vi "Get Channel Attribute Double Wrapper.vi"(0 "Task map in":map{string, refnum<k21>}(c390), 5 "Message Data in":T2, 11 "error in (no error)":errorcluster) -> (4 "Task map out":map{string, refnum<k21>}(c390), 6 "Message Data out":T1, 15 "error out":errorcluster)   [LabVIEW 2021, in "NI DAQmx_wrapper.lvlib"]
uses:
  NI DAQmx_wrapper.lvlib
  NI DAQmx_server/RPC Messages/nidaqmx_grpc_GetChanAttributeDoubleRequest.ctl
  NI DAQmx_server/RPC Messages/nidevice_grpc_Session_session/nidevice_grpc_Session_session.lvclass
  NI DAQmx_server/RPC Messages/nidaqmx_grpc_GetChanAttributeDoubleRequest_attribute_enum/nidaqmx_grpc_GetChanAttributeDoubleRequest_attribute_enum.lvclass
  NI DAQmx_server/RPC Messages/nidevice_grpc_Session.ctl
  NI DAQmx_server/RPC Messages/nidaqmx_grpc_GetChanAttributeDoubleResponse.ctl
  NI DAQmx_server/RPC Messages/nidaqmx_grpc_GetChanAttributeDoubleRequest_attribute_enum/nidaqmx_grpc_GetChanAttributeDoubleRequest_attribute_enum.lvclass/nidaqmx_grpc_GetChanAttributeDoubleRequest_attribute_enum.ctl
  NI DAQmx_server/RPC Messages/nidevice_grpc_Session_session/nidevice_grpc_Session_session.lvclass/nidevice_grpc_Session_session.ctl
  <resource>/objmgr/daqmx.rc
  NI DAQmx_server/NI DAQmx_server.lvlib
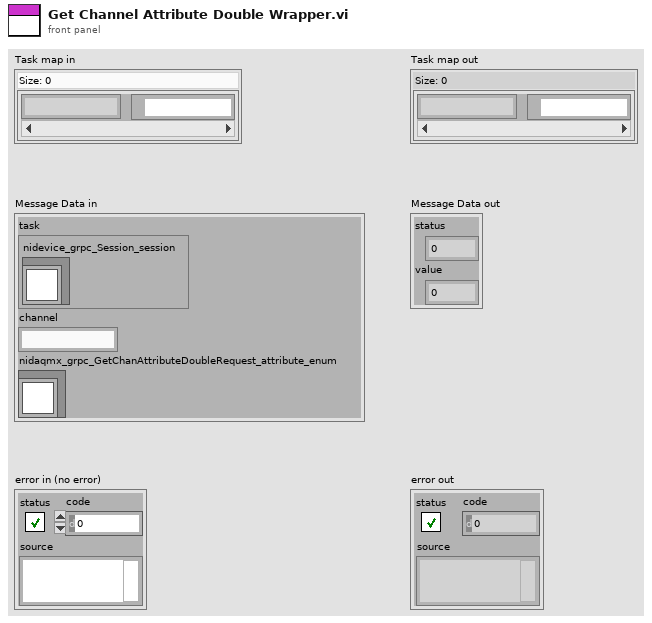
[diagram p1: front panel]
types:
  T1 = typedef "NI DAQmx_server.lvlib/nidaqmx_grpc_GetChanAttributeDoubleResponse.ctl" = cluster{"status":i32, "value":dbl}
  T2 = typedef "NI DAQmx_server.lvlib/nidaqmx_grpc_GetChanAttributeDoubleRequest.ctl" = cluster{"task":T3, "channel":string, "nidaqmx_grpc_GetChanAttributeDoubleRequest_attribute_enum":refnum<class "nidaqmx_grpc_GetChanAttributeDoubleRequest_attribute_enum.lvclass">}
  T3 = typedef "NI DAQmx_server.lvlib/nidevice_grpc_Session.ctl" = cluster{"nidevice_grpc_Session_session":refnum<class "nidevice_grpc_Session_session.lvclass">}
  T4 = typedef "NI DAQmx_server.lvlib/nidaqmx_grpc_ChannelDoubleAttribute.ctl" = enum32{"CHANNEL_DOUBLE_ATTRIBUTE_UNSPECIFIED", "CHANNEL_ATTRIBUTE_AI_IMPEDANCE", "CHANNEL_ATTRIBUTE_AI_AC_EXCIT_FREQ", "CHANNEL_ATTRIBUTE_AO_GAIN", "CHANNEL_ATTRIBUTE_AO_LOAD_IMPEDANCE", "CHANNEL_ATTRIBUTE_CI_FREQ_MEAS_TIME", "CHANNEL_ATTRIBUTE_CO_PULSE_FREQ_INITIAL_DELAY", "CHANNEL_ATTRIBUTE_AI_ACCEL_SENSITIVITY", "CHANNEL_ATTRIBUTE_AI_FREQ_HYST", "CHANNEL_ATTRIBUTE_AI_FREQ_THRESH_VOLTAGE", "CHANNEL_ATTRIBUTE_CI_ANG_ENCODER_INITIAL_ANGLE", "CHANNEL_ATTRIBUTE_CI_ENCODER_Z_INDEX_VAL", "CHANNEL_ATTRIBUTE_AI_RVDT_SENSITIVITY", "CHANNEL_ATTRIBUTE_CI_LIN_ENCODER_DIST_PER_PULSE", "CHANNEL_ATTRIBUTE_CI_LIN_ENCODER_INITIAL_POS", "CHANNEL_ATTRIBUTE_AI_LVDT_SENSITIVITY", "CHANNEL_ATTRIBUTE_AI_STRAIN_GAGE_GAGE_FACTOR", "CHANNEL_ATTRIBUTE_AI_STRAIN_GAGE_POISSON_RATIO", "CHANNEL_ATTRIBUTE_AI_RTD_A", "CHANNEL_ATTRIBUTE_AI_RTD_B", "CHANNEL_ATTRIBUTE_AI_RTD_C", "CHANNEL_ATTRIBUTE_AI_RTD_R0", "CHANNEL_ATTRIBUTE_AI_THRMCPL_CJC_VAL", "CHANNEL_ATTRIBUTE_AI_THRMSTR_R1", "CHANNEL_ATTRIBUTE_CO_PULSE_DUTY_CYC", "CHANNEL_ATTRIBUTE_CO_PULSE_FREQ", "CHANNEL_ATTRIBUTE_AO_MAX", "CHANNEL_ATTRIBUTE_AO_MIN", "CHANNEL_ATTRIBUTE_AO_OUTPUT_IMPEDANCE", "CHANNEL_ATTRIBUTE_AI_MICROPHONE_SENSITIVITY", "CHANNEL_ATTRIBUTE_AI_RESOLUTION", "CHANNEL_ATTRIBUTE_AI_MAX", "CHANNEL_ATTRIBUTE_AI_MIN", "CHANNEL_ATTRIBUTE_AI_BRIDGE_NOM_RESISTANCE", "CHANNEL_ATTRIBUTE_AI_BRIDGE_INITIAL_VOLTAGE", "CHANNEL_ATTRIBUTE_AI_LEAD_WIRE_RESISTANCE", "CHANNEL_ATTRIBUTE_AI_CURRENT_SHUNT_RESISTANCE", "CHANNEL_ATTRIBUTE_AI_EXCIT_VAL", "CHANNEL_ATTRIBUTE_AI_ATTEN", "CHANNEL_ATTRIBUTE_AI_LOWPASS_CUTOFF_FREQ", "CHANNEL_ATTRIBUTE_AI_HIGHPASS_CUTOFF_FREQ", "CHANNEL_ATTRIBUTE_AI_BANDPASS_CENTER_FREQ", "CHANNEL_ATTRIBUTE_AI_BANDPASS_WIDTH", "CHANNEL_ATTRIBUTE_AI_NOTCH_CENTER_FREQ", "CHANNEL_ATTRIBUTE_AI_NOTCH_WIDTH", "CHANNEL_ATTRIBUTE_AI_RNG_HIGH", "CHANNEL_ATTRIBUTE_AI_RNG_LOW", "CHANNEL_ATTRIBUTE_AI_GAIN", "CHANNEL_ATTRIBUTE_AO_RESOLUTION", "CHANNEL_ATTRIBUTE_AO_DAC_RNG_LOW", "CHANNEL_ATTRIBUTE_AO_DAC_RNG_HIGH", "CHANNEL_ATTRIBUTE_AO_DAC_REF_VAL", "CHANNEL_ATTRIBUTE_AI_EXCIT_ACTUAL_VAL", "CHANNEL_ATTRIBUTE_AI_LOWPASS_SWITCH_CAP_EXT_CLK_FREQ", "CHANNEL_ATTRIBUTE_CI_MAX", "CHANNEL_ATTRIBUTE_CI_MIN", "CHANNEL_ATTRIBUTE_CI_CTR_TIMEBASE_RATE", "CHANNEL_ATTRIBUTE_CO_PULSE_HIGH_TIME", "CHANNEL_ATTRIBUTE_CO_PULSE_LOW_TIME", "CHANNEL_ATTRIBUTE_CO_PULSE_TIME_INITIAL_DELAY", "CHANNEL_ATTRIBUTE_CO_CTR_TIMEBASE_RATE", "CHANNEL_ATTRIBUTE_AI_THRMSTR_A", "CHANNEL_ATTRIBUTE_AI_THRMSTR_C", "CHANNEL_ATTRIBUTE_AI_THRMSTR_B", "CHANNEL_ATTRIBUTE_CI_PERIOD_MEAS_TIME", "CHANNEL_ATTRIBUTE_AI_BRIDGE_SHUNT_CAL_GAIN_ADJUST", "CHANNEL_ATTRIBUTE_DI_DIG_FLTR_MIN_PULSE_WIDTH", "CHANNEL_ATTRIBUTE_CI_FREQ_DIG_FLTR_MIN_PULSE_WIDTH", "CHANNEL_ATTRIBUTE_CI_FREQ_DIG_FLTR_TIMEBASE_RATE", "CHANNEL_ATTRIBUTE_CI_PERIOD_DIG_FLTR_MIN_PULSE_WIDTH", "CHANNEL_ATTRIBUTE_CI_PERIOD_DIG_FLTR_TIMEBASE_RATE", "CHANNEL_ATTRIBUTE_CI_COUNT_EDGES_COUNT_DIR_DIG_FLTR_MIN_PULSE_WIDTH", "CHANNEL_ATTRIBUTE_CI_COUNT_EDGES_COUNT_DIR_DIG_FLTR_TIMEBASE_RATE", "CHANNEL_ATTRIBUTE_CI_COUNT_EDGES_DIG_FLTR_MIN_PULSE_WIDTH", "CHANNEL_ATTRIBUTE_CI_COUNT_EDGES_DIG_FLTR_TIMEBASE_RATE", "CHANNEL_ATTRIBUTE_CI_ENCODER_A_INPUT_DIG_FLTR_MIN_PULSE_WIDTH", "CHANNEL_ATTRIBUTE_CI_ENCODER_A_INPUT_DIG_FLTR_TIMEBASE_RATE", "CHANNEL_ATTRIBUTE_CI_ENCODER_B_INPUT_DIG_FLTR_MIN_PULSE_WIDTH", "CHANNEL_ATTRIBUTE_CI_ENCODER_B_INPUT_DIG_FLTR_TIMEBASE_RATE", "CHANNEL_ATTRIBUTE_CI_ENCODER_Z_INPUT_DIG_FLTR_MIN_PULSE_WIDTH", "CHANNEL_ATTRIBUTE_CI_ENCODER_Z_INPUT_DIG_FLTR_TIMEBASE_RATE", "CHANNEL_ATTRIBUTE_CI_PULSE_WIDTH_DIG_FLTR_MIN_PULSE_WIDTH", "CHANNEL_ATTRIBUTE_CI_PULSE_WIDTH_DIG_FLTR_TIMEBASE_RATE", "CHANNEL_ATTRIBUTE_CI_TWO_EDGE_SEP_FIRST_DIG_FLTR_MIN_PULSE_WIDTH", "CHANNEL_ATTRIBUTE_CI_TWO_EDGE_SEP_FIRST_DIG_FLTR_TIMEBASE_RATE", "CHANNEL_ATTRIBUTE_CI_TWO_EDGE_SEP_SECOND_DIG_FLTR_MIN_PULSE_WIDTH", "CHANNEL_ATTRIBUTE_CI_TWO_EDGE_SEP_SECOND_DIG_FLTR_TIMEBASE_RATE", "CHANNEL_ATTRIBUTE_CI_SEMI_PERIOD_DIG_FLTR_MIN_PULSE_WIDTH", "CHANNEL_ATTRIBUTE_CI_SEMI_PERIOD_DIG_FLTR_TIMEBASE_RATE", "CHANNEL_ATTRIBUTE_AI_SOUND_PRESSURE_MAX_SOUND_PRESSURE_LVL", "CHANNEL_ATTRIBUTE_AO_DAC_OFFSET_VAL", "CHANNEL_ATTRIBUTE_CI_CTR_TIMEBASE_DIG_FLTR_MIN_PULSE_WIDTH", "CHANNEL_ATTRIBUTE_CI_CTR_TIMEBASE_DIG_FLTR_TIMEBASE_RATE", "CHANNEL_ATTRIBUTE_CO_CTR_TIMEBASE_DIG_FLTR_MIN_PULSE_WIDTH", "CHANNEL_ATTRIBUTE_CO_CTR_TIMEBASE_DIG_FLTR_TIMEBASE_RATE", "CHANNEL_ATTRIBUTE_AI_VOLTAGE_DB_REF", "CHANNEL_ATTRIBUTE_AI_SOUND_PRESSURE_DB_REF", "CHANNEL_ATTRIBUTE_AI_ACCEL_DB_REF", "CHANNEL_ATTRIBUTE_AO_FUNC_GEN_FREQ", "CHANNEL_ATTRIBUTE_AO_FUNC_GEN_AMPLITUDE", "CHANNEL_ATTRIBUTE_AO_FUNC_GEN_OFFSET", "CHANNEL_ATTRIBUTE_AO_FUNC_GEN_SQUARE_DUTY_CYCLE", "CHANNEL_ATTRIBUTE_AO_VOLTAGE_CURRENT_LIMIT", "CHANNEL_ATTRIBUTE_AO_FUNC_GEN_FM_DEVIATION", "CHANNEL_ATTRIBUTE_DO_OVERCURRENT_LIMIT", "CHANNEL_ATTRIBUTE_DO_OVERCURRENT_REENABLE_PERIOD", "CHANNEL_ATTRIBUTE_AI_PROBE_ATTEN", "CHANNEL_ATTRIBUTE_AI_DC_OFFSET", "CHANNEL_ATTRIBUTE_AI_EDDY_CURRENT_PROX_PROBE_SENSITIVITY", "CHANNEL_ATTRIBUTE_DI_DIG_FLTR_TIMEBASE_RATE", "CHANNEL_ATTRIBUTE_CI_PULSE_FREQ_DIG_FLTR_MIN_PULSE_WIDTH", "CHANNEL_ATTRIBUTE_CI_PULSE_FREQ_DIG_FLTR_TIMEBASE_RATE", "CHANNEL_ATTRIBUTE_CI_PULSE_TIME_DIG_FLTR_MIN_PULSE_WIDTH", "CHANNEL_ATTRIBUTE_CI_PULSE_TIME_DIG_FLTR_TIMEBASE_RATE", "CHANNEL_ATTRIBUTE_CI_PULSE_TICKS_DIG_FLTR_MIN_PULSE_WIDTH", "CHANNEL_ATTRIBUTE_CI_PULSE_TICKS_DIG_FLTR_TIMEBASE_RATE", "CHANNEL_ATTRIBUTE_AI_BRIDGE_SHUNT_CAL_SHUNT_CAL_A_RESISTANCE", "CHANNEL_ATTRIBUTE_AI_BRIDGE_SHUNT_CAL_SHUNT_CAL_A_ACTUAL_RESISTANCE", "CHANNEL_ATTRIBUTE_AI_BRIDGE_SHUNT_CAL_SHUNT_CAL_B_RESISTANCE", "CHANNEL_ATTRIBUTE_AI_BRIDGE_SHUNT_CAL_SHUNT_CAL_B_ACTUAL_RESISTANCE", "CHANNEL_ATTRIBUTE_AI_FORCE_IEPE_SENSOR_SENSITIVITY", "CHANNEL_ATTRIBUTE_AI_BRIDGE_INITIAL_RATIO", "CHANNEL_ATTRIBUTE_AI_BRIDGE_TWO_POINT_LIN_FIRST_ELECTRICAL_VAL", "CHANNEL_ATTRIBUTE_AI_BRIDGE_TWO_POINT_LIN_FIRST_PHYSICAL_VAL", "CHANNEL_ATTRIBUTE_AI_BRIDGE_TWO_POINT_LIN_SECOND_ELECTRICAL_VAL", "CHANNEL_ATTRIBUTE_AI_BRIDGE_TWO_POINT_LIN_SECOND_PHYSICAL_VAL", "CHANNEL_ATTRIBUTE_CI_COUNT_EDGES_COUNT_RESET_DIG_FLTR_MIN_PULSE_WIDTH", "CHANNEL_ATTRIBUTE_CI_COUNT_EDGES_COUNT_RESET_DIG_FLTR_TIMEBASE_RATE", "CHANNEL_ATTRIBUTE_AI_THRMCPL_LEAD_OFFSET_VOLTAGE", "CHANNEL_ATTRIBUTE_AI_FILTER_DELAY", "CHANNEL_ATTRIBUTE_AI_VELOCITY_IEPE_SENSOR_DB_REF", "CHANNEL_ATTRIBUTE_AI_VELOCITY_IEPE_SENSOR_SENSITIVITY", "CHANNEL_ATTRIBUTE_AI_ROSETTE_STRAIN_GAGE_ORIENTATION", "CHANNEL_ATTRIBUTE_AO_FILTER_DELAY_ADJUSTMENT", "CHANNEL_ATTRIBUTE_AI_FILTER_DELAY_ADJUSTMENT", "CHANNEL_ATTRIBUTE_AO_FILTER_DELAY", "CHANNEL_ATTRIBUTE_CI_DUTY_CYCLE_DIG_FLTR_MIN_PULSE_WIDTH", "CHANNEL_ATTRIBUTE_CI_DUTY_CYCLE_DIG_FLTR_TIMEBASE_RATE", "CHANNEL_ATTRIBUTE_CI_MAX_MEAS_PERIOD", "CHANNEL_ATTRIBUTE_CI_THRESH_VOLTAGE", "CHANNEL_ATTRIBUTE_AI_DIG_FLTR_LOWPASS_CUTOFF_FREQ", "CHANNEL_ATTRIBUTE_AI_DIG_FLTR_HIGHPASS_CUTOFF_FREQ", "CHANNEL_ATTRIBUTE_AI_DIG_FLTR_BANDPASS_CENTER_FREQ", "CHANNEL_ATTRIBUTE_AI_DIG_FLTR_BANDPASS_WIDTH", "CHANNEL_ATTRIBUTE_AI_DIG_FLTR_NOTCH_CENTER_FREQ", "CHANNEL_ATTRIBUTE_AI_DIG_FLTR_NOTCH_WIDTH", "CHANNEL_ATTRIBUTE_CI_VELOCITY_LIN_ENCODER_DIST_PER_PULSE", "CHANNEL_ATTRIBUTE_CI_VELOCITY_ENCODER_A_INPUT_DIG_FLTR_MIN_PULSE_WIDTH", "CHANNEL_ATTRIBUTE_CI_VELOCITY_ENCODER_A_INPUT_DIG_FLTR_TIMEBASE_RATE", "CHANNEL_ATTRIBUTE_CI_VELOCITY_ENCODER_B_INPUT_DIG_FLTR_MIN_PULSE_WIDTH", "CHANNEL_ATTRIBUTE_CI_VELOCITY_ENCODER_B_INPUT_DIG_FLTR_TIMEBASE_RATE", "CHANNEL_ATTRIBUTE_CI_VELOCITY_MEAS_TIME", "CHANNEL_ATTRIBUTE_CI_COUNT_EDGES_GATE_DIG_FLTR_MIN_PULSE_WIDTH", "CHANNEL_ATTRIBUTE_CI_COUNT_EDGES_GATE_DIG_FLTR_TIMEBASE_RATE", "CHANNEL_ATTRIBUTE_AI_ACCEL_CHARGE_SENSITIVITY", "CHANNEL_ATTRIBUTE_AI_ACCEL_4_WIRE_DC_VOLTAGE_SENSITIVITY", "CHANNEL_ATTRIBUTE_AI_DATA_XFER_MAX_RATE", "CHANNEL_ATTRIBUTE_AI_SENSOR_POWER_VOLTAGE", "CHANNEL_ATTRIBUTE_AI_FILTER_FREQ", "CHANNEL_ATTRIBUTE_AI_INPUT_LIMITS_FAULT_DETECT_UPPER_LIMIT", "CHANNEL_ATTRIBUTE_AI_INPUT_LIMITS_FAULT_DETECT_LOWER_LIMIT", "CHANNEL_ATTRIBUTE_CI_FREQ_THRESH_VOLTAGE", "CHANNEL_ATTRIBUTE_CI_FREQ_HYST", "CHANNEL_ATTRIBUTE_CI_PERIOD_THRESH_VOLTAGE", "CHANNEL_ATTRIBUTE_CI_PERIOD_HYST", "CHANNEL_ATTRIBUTE_CI_COUNT_EDGES_THRESH_VOLTAGE", "CHANNEL_ATTRIBUTE_CI_COUNT_EDGES_HYST", "CHANNEL_ATTRIBUTE_CI_COUNT_EDGES_COUNT_DIR_THRESH_VOLTAGE", "CHANNEL_ATTRIBUTE_CI_COUNT_EDGES_COUNT_DIR_HYST", "CHANNEL_ATTRIBUTE_CI_COUNT_EDGES_COUNT_RESET_THRESH_VOLTAGE", "CHANNEL_ATTRIBUTE_CI_COUNT_EDGES_COUNT_RESET_HYST", "CHANNEL_ATTRIBUTE_CI_COUNT_EDGES_GATE_THRESH_VOLTAGE", "CHANNEL_ATTRIBUTE_CI_COUNT_EDGES_GATE_HYST", "CHANNEL_ATTRIBUTE_CI_FILTER_FREQ", "CHANNEL_ATTRIBUTE_CI_FILTER_DELAY", "CHANNEL_ATTRIBUTE_AO_FUNC_GEN_START_PHASE", "CHANNEL_ATTRIBUTE_AO_COMMON_MODE_OFFSET", "CHANNEL_ATTRIBUTE_PWR_VOLTAGE_SETPOINT", "CHANNEL_ATTRIBUTE_PWR_CURRENT_SETPOINT"}
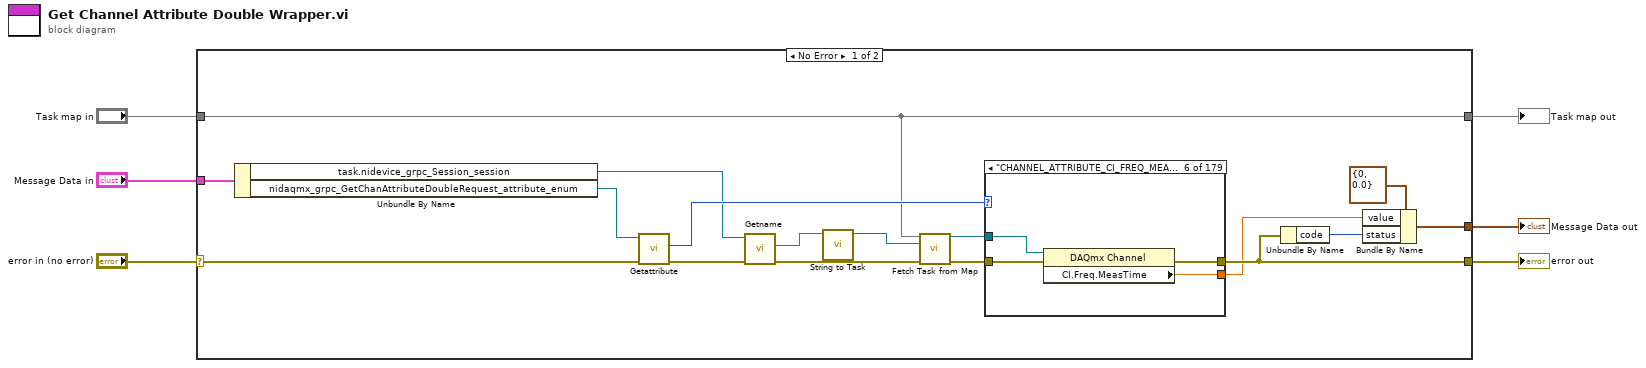
[diagram p0: block diagram]
diagram:
  n1 = case shown="No Error" "error in (no error)" {
    selector: "error in (no error)" -> [w22 w207]
    tunnel: [w10 w207] -> w5
    tunnel: "Task map in" -> [w13 w206]
    tunnel: [w13 w206] -> w3
    tunnel: "Message Data in" -> [w23 _]
    tunnel: [w7 _] -> w1
    frame No Error {
      n2 = Unbundle By Name(w23) -> ("task.nidevice_grpc_Session_session"=w14:refnum<class "nidevice_grpc_Session_session.lvclass">, "nidaqmx_grpc_GetChanAttributeDoubleRequest_attribute_enum"=w21:refnum<class "nidaqmx_grpc_GetChanAttributeDoubleRequest_attribute_enum.lvclass">)
      n3 = call "Getattribute.vi"("error in (no error)"=w22, "OneOfTemplate in"=w21) -> ("error out"=w16:errorcluster, "Get_Val"=w20:T4)  [unwired: 7 in, 1 out]
      n4 = call "Getname.vi"("error in (no error)"=w16, "OneOfTemplate in"=w14) -> ("error out"=w17:errorcluster, "Get_Val"=w19:string)  [unwired: 7 in, 1 out]
      n5 = call "String to Task.vi"("Get_Val"=w19) -> ("Refnum out"=w18:refnum<k21>)  [unwired: 10 in]
      n6 = call "Fetch Task from Map.vi"("Task map in"=w13, "Task in"=w18, "error in (no error)"=w17) -> ("Task out"=w12:refnum<k21>, "error out"=w15:errorcluster)  [unwired: 11 in]
      n7 = case shown="\"CHANNEL_ATTRIBUTE_CI_FREQ_MEAS_TIME\"" w20 {
        tunnel: w15 -> [w24 w25 w26 w27 w28 w32 w33 w34 w35 w36 w37 w38 w39 w40 w41 w42 w43 w44 w45 w46 w47 w48 w49 w50 w51 w52 w53 w54 w55 w56 w57 w58 w59 w60 w61 w62 w63 w64 w65 w66 w67 w68 w69 w70 w71 w72 w73 w74 w75 w76 w77 w78 w79 w80 w81 w82 w83 w84 w85 w86 w87 w88 w89 w90 w91 w92 w93 w94 w95 w96 w97 w98 w99 w100 w101 w102 w103 w104 w105 w106 w107 w108 w109 w110 w111 w112 w113 w114 w115 w116 w117 w118 w119 w120 w121 w122 w123 w124 w125 w126 w127 w128 w129 w130 w131 w132 w133 w134 w135 w136 w137 w138 w139 w140 w141 w142 w143 w144 w145 w146 w147 w148 w149 w150 w151 w152 w153 w154 w155 w156 w157 w158 w159 w160 w161 w162 w163 w164 w165 w166 w167 w168 w169 w170 w171 w172 w173 w174 w175 w176 w177 w178 w179 w180 w181 w182 w183 w184 w185 w186 w187 w188 w189 w190 w191 w192 w193 w194 w195 w196 w197 w198 w199 w200 w201 w202 w203 w204 w205]
        tunnel: [w24 w25 w26 w27 w28 w31 w33 w34 w35 w36 w37 w38 w39 w40 w41 w42 w43 w44 w45 w46 w47 w48 w49 w50 w51 w52 w53 w54 w55 w56 w57 w58 w59 w60 w61 w62 w63 w64 w65 w66 w67 w68 w69 w70 w71 w72 w73 w74 w75 w76 w77 w78 w79 w80 w81 w82 w83 w84 w85 w86 w87 w88 w89 w90 w91 w92 w93 w94 w95 w96 w97 w98 w99 w100 w101 w102 w103 w104 w105 w106 w107 w108 w109 w110 w111 w112 w113 w114 w115 w116 w117 w118 w119 w120 w121 w122 w123 w124 w125 w126 w127 w128 w129 w130 w131 w132 w133 w134 w135 w136 w137 w138 w139 w140 w141 w142 w143 w144 w145 w146 w147 w148 w149 w150 w151 w152 w153 w154 w155 w156 w157 w158 w159 w160 w161 w162 w163 w164 w165 w166 w167 w168 w169 w170 w171 w172 w173 w174 w175 w176 w177 w178 w179 w180 w181 w182 w183 w184 w185 w186 w187 w188 w189 w190 w191 w192 w193 w194 w195 w196 w197 w198 w199 w200 w201 w202 w203 w204 w205] -> w10
        tunnel: w12 -> [_ _ _ _ _ w30 _ _ _ _ _ _ _ _ _ _ _ _ _ _ _ _ _ _ _ _ _ _ _ _ _ _ _ _ _ _ _ _ _ _ _ _ _ _ _ _ _ _ _ _ _ _ _ _ _ _ _ _ _ _ _ _ _ _ _ _ _ _ _ _ _ _ _ _ _ _ _ _ _ _ _ _ _ _ _ _ _ _ _ _ _ _ _ _ _ _ _ _ _ _ _ _ _ _ _ _ _ _ _ _ _ _ _ _ _ _ _ _ _ _ _ _ _ _ _ _ _ _ _ _ _ _ _ _ _ _ _ _ _ _ _ _ _ _ _ _ _ _ _ _ _ _ _ _ _ _ _ _ _ _ _ _ _ _ _ _ _ _ _ _ _ _ _ _ _ _ _ _ _]
        tunnel: [_ _ _ _ _ w29 _ _ _ _ _ _ _ _ _ _ _ _ _ _ _ _ _ _ _ _ _ _ _ _ _ _ _ _ _ _ _ _ _ _ _ _ _ _ _ _ _ _ _ _ _ _ _ _ _ _ _ _ _ _ _ _ _ _ _ _ _ _ _ _ _ _ _ _ _ _ _ _ _ _ _ _ _ _ _ _ _ _ _ _ _ _ _ _ _ _ _ _ _ _ _ _ _ _ _ _ _ _ _ _ _ _ _ _ _ _ _ _ _ _ _ _ _ _ _ _ _ _ _ _ _ _ _ _ _ _ _ _ _ _ _ _ _ _ _ _ _ _ _ _ _ _ _ _ _ _ _ _ _ _ _ _ _ _ _ _ _ _ _ _ _ _ _ _ _ _ _ _ _] -> w8
        frame "CHANNEL_DOUBLE_ATTRIBUTE_UNSPECIFIED", Default {
        }
        frame "CHANNEL_ATTRIBUTE_AI_IMPEDANCE" {
        }
        frame "CHANNEL_ATTRIBUTE_AI_AC_EXCIT_FREQ" {
        }
        frame "CHANNEL_ATTRIBUTE_AO_GAIN" {
        }
        frame "CHANNEL_ATTRIBUTE_AO_LOAD_IMPEDANCE" {
        }
        frame "CHANNEL_ATTRIBUTE_CI_FREQ_MEAS_TIME" {
          n8 = property class="DAQmx Channel"(reference=w30, error in=w32) -> (error out=w31:errorcluster, "CI.Freq.MeasTime"=w29:dbl)  [unwired: 1 out]
        }
        frame "CHANNEL_ATTRIBUTE_CO_PULSE_FREQ_INITIAL_DELAY" {
        }
        frame "CHANNEL_ATTRIBUTE_AI_ACCEL_SENSITIVITY" {
        }
        frame "CHANNEL_ATTRIBUTE_AI_FREQ_HYST" {
        }
        frame "CHANNEL_ATTRIBUTE_AI_FREQ_THRESH_VOLTAGE" {
        }
        frame "CHANNEL_ATTRIBUTE_CI_ANG_ENCODER_INITIAL_ANGLE" {
        }
        frame "CHANNEL_ATTRIBUTE_CI_ENCODER_Z_INDEX_VAL" {
        }
        frame "CHANNEL_ATTRIBUTE_AI_RVDT_SENSITIVITY" {
        }
        frame "CHANNEL_ATTRIBUTE_CI_LIN_ENCODER_DIST_PER_PULSE" {
        }
        frame "CHANNEL_ATTRIBUTE_CI_LIN_ENCODER_INITIAL_POS" {
        }
        frame "CHANNEL_ATTRIBUTE_AI_LVDT_SENSITIVITY" {
        }
        frame "CHANNEL_ATTRIBUTE_AI_STRAIN_GAGE_GAGE_FACTOR" {
        }
        frame "CHANNEL_ATTRIBUTE_AI_STRAIN_GAGE_POISSON_RATIO" {
        }
        frame "CHANNEL_ATTRIBUTE_AI_RTD_A" {
        }
        frame "CHANNEL_ATTRIBUTE_AI_RTD_B" {
        }
        frame "CHANNEL_ATTRIBUTE_AI_RTD_C" {
        }
        frame "CHANNEL_ATTRIBUTE_AI_RTD_R0" {
        }
        frame "CHANNEL_ATTRIBUTE_AI_THRMCPL_CJC_VAL" {
        }
        frame "CHANNEL_ATTRIBUTE_AI_THRMSTR_R1" {
        }
        frame "CHANNEL_ATTRIBUTE_CO_PULSE_DUTY_CYC" {
        }
        frame "CHANNEL_ATTRIBUTE_CO_PULSE_FREQ" {
        }
        frame "CHANNEL_ATTRIBUTE_AO_MAX" {
        }
        frame "CHANNEL_ATTRIBUTE_AO_MIN" {
        }
        frame "CHANNEL_ATTRIBUTE_AO_OUTPUT_IMPEDANCE" {
        }
        frame "CHANNEL_ATTRIBUTE_AI_MICROPHONE_SENSITIVITY" {
        }
        frame "CHANNEL_ATTRIBUTE_AI_RESOLUTION" {
        }
        frame "CHANNEL_ATTRIBUTE_AI_MAX" {
        }
        frame "CHANNEL_ATTRIBUTE_AI_MIN" {
        }
        frame "CHANNEL_ATTRIBUTE_AI_BRIDGE_NOM_RESISTANCE" {
        }
        frame "CHANNEL_ATTRIBUTE_AI_BRIDGE_INITIAL_VOLTAGE" {
        }
        frame "CHANNEL_ATTRIBUTE_AI_LEAD_WIRE_RESISTANCE" {
        }
        frame "CHANNEL_ATTRIBUTE_AI_CURRENT_SHUNT_RESISTANCE" {
        }
        frame "CHANNEL_ATTRIBUTE_AI_EXCIT_VAL" {
        }
        frame "CHANNEL_ATTRIBUTE_AI_ATTEN" {
        }
        frame "CHANNEL_ATTRIBUTE_AI_LOWPASS_CUTOFF_FREQ" {
        }
        frame "CHANNEL_ATTRIBUTE_AI_HIGHPASS_CUTOFF_FREQ" {
        }
        frame "CHANNEL_ATTRIBUTE_AI_BANDPASS_CENTER_FREQ" {
        }
        frame "CHANNEL_ATTRIBUTE_AI_BANDPASS_WIDTH" {
        }
        frame "CHANNEL_ATTRIBUTE_AI_NOTCH_CENTER_FREQ" {
        }
        frame "CHANNEL_ATTRIBUTE_AI_NOTCH_WIDTH" {
        }
        frame "CHANNEL_ATTRIBUTE_AI_RNG_HIGH" {
        }
        frame "CHANNEL_ATTRIBUTE_AI_RNG_LOW" {
        }
        frame "CHANNEL_ATTRIBUTE_AI_GAIN" {
        }
        frame "CHANNEL_ATTRIBUTE_AO_RESOLUTION" {
        }
        frame "CHANNEL_ATTRIBUTE_AO_DAC_RNG_LOW" {
        }
        frame "CHANNEL_ATTRIBUTE_AO_DAC_RNG_HIGH" {
        }
        frame "CHANNEL_ATTRIBUTE_AO_DAC_REF_VAL" {
        }
        frame "CHANNEL_ATTRIBUTE_AI_EXCIT_ACTUAL_VAL" {
        }
        frame "CHANNEL_ATTRIBUTE_AI_LOWPASS_SWITCH_CAP_EXT_CLK_FREQ" {
        }
        frame "CHANNEL_ATTRIBUTE_CI_MAX" {
        }
        frame "CHANNEL_ATTRIBUTE_CI_MIN" {
        }
        frame "CHANNEL_ATTRIBUTE_CI_CTR_TIMEBASE_RATE" {
        }
        frame "CHANNEL_ATTRIBUTE_CO_PULSE_HIGH_TIME" {
        }
        frame "CHANNEL_ATTRIBUTE_CO_PULSE_LOW_TIME" {
        }
        frame "CHANNEL_ATTRIBUTE_CO_PULSE_TIME_INITIAL_DELAY" {
        }
        frame "CHANNEL_ATTRIBUTE_CO_CTR_TIMEBASE_RATE" {
        }
        frame "CHANNEL_ATTRIBUTE_AI_THRMSTR_A" {
        }
        frame "CHANNEL_ATTRIBUTE_AI_THRMSTR_C" {
        }
        frame "CHANNEL_ATTRIBUTE_AI_THRMSTR_B" {
        }
        frame "CHANNEL_ATTRIBUTE_CI_PERIOD_MEAS_TIME" {
        }
        frame "CHANNEL_ATTRIBUTE_AI_BRIDGE_SHUNT_CAL_GAIN_ADJUST" {
        }
        frame "CHANNEL_ATTRIBUTE_DI_DIG_FLTR_MIN_PULSE_WIDTH" {
        }
        frame "CHANNEL_ATTRIBUTE_CI_FREQ_DIG_FLTR_MIN_PULSE_WIDTH" {
        }
        frame "CHANNEL_ATTRIBUTE_CI_FREQ_DIG_FLTR_TIMEBASE_RATE" {
        }
        frame "CHANNEL_ATTRIBUTE_CI_PERIOD_DIG_FLTR_MIN_PULSE_WIDTH" {
        }
        frame "CHANNEL_ATTRIBUTE_CI_PERIOD_DIG_FLTR_TIMEBASE_RATE" {
        }
        frame "CHANNEL_ATTRIBUTE_CI_COUNT_EDGES_COUNT_DIR_DIG_FLTR_MIN_PULSE_WIDTH" {
        }
        frame "CHANNEL_ATTRIBUTE_CI_COUNT_EDGES_COUNT_DIR_DIG_FLTR_TIMEBASE_RATE" {
        }
        frame "CHANNEL_ATTRIBUTE_CI_COUNT_EDGES_DIG_FLTR_MIN_PULSE_WIDTH" {
        }
        frame "CHANNEL_ATTRIBUTE_CI_COUNT_EDGES_DIG_FLTR_TIMEBASE_RATE" {
        }
        frame "CHANNEL_ATTRIBUTE_CI_ENCODER_A_INPUT_DIG_FLTR_MIN_PULSE_WIDTH" {
        }
        frame "CHANNEL_ATTRIBUTE_CI_ENCODER_A_INPUT_DIG_FLTR_TIMEBASE_RATE" {
        }
        frame "CHANNEL_ATTRIBUTE_CI_ENCODER_B_INPUT_DIG_FLTR_MIN_PULSE_WIDTH" {
        }
        frame "CHANNEL_ATTRIBUTE_CI_ENCODER_B_INPUT_DIG_FLTR_TIMEBASE_RATE" {
        }
        frame "CHANNEL_ATTRIBUTE_CI_ENCODER_Z_INPUT_DIG_FLTR_MIN_PULSE_WIDTH" {
        }
        frame "CHANNEL_ATTRIBUTE_CI_ENCODER_Z_INPUT_DIG_FLTR_TIMEBASE_RATE" {
        }
        frame "CHANNEL_ATTRIBUTE_CI_PULSE_WIDTH_DIG_FLTR_MIN_PULSE_WIDTH" {
        }
        frame "CHANNEL_ATTRIBUTE_CI_PULSE_WIDTH_DIG_FLTR_TIMEBASE_RATE" {
        }
        frame "CHANNEL_ATTRIBUTE_CI_TWO_EDGE_SEP_FIRST_DIG_FLTR_MIN_PULSE_WIDTH" {
        }
        frame "CHANNEL_ATTRIBUTE_CI_TWO_EDGE_SEP_FIRST_DIG_FLTR_TIMEBASE_RATE" {
        }
        frame "CHANNEL_ATTRIBUTE_CI_TWO_EDGE_SEP_SECOND_DIG_FLTR_MIN_PULSE_WIDTH" {
        }
        frame "CHANNEL_ATTRIBUTE_CI_TWO_EDGE_SEP_SECOND_DIG_FLTR_TIMEBASE_RATE" {
        }
        frame "CHANNEL_ATTRIBUTE_CI_SEMI_PERIOD_DIG_FLTR_MIN_PULSE_WIDTH" {
        }
        frame "CHANNEL_ATTRIBUTE_CI_SEMI_PERIOD_DIG_FLTR_TIMEBASE_RATE" {
        }
        frame "CHANNEL_ATTRIBUTE_AI_SOUND_PRESSURE_MAX_SOUND_PRESSURE_LVL" {
        }
        frame "CHANNEL_ATTRIBUTE_AO_DAC_OFFSET_VAL" {
        }
        frame "CHANNEL_ATTRIBUTE_CI_CTR_TIMEBASE_DIG_FLTR_MIN_PULSE_WIDTH" {
        }
        frame "CHANNEL_ATTRIBUTE_CI_CTR_TIMEBASE_DIG_FLTR_TIMEBASE_RATE" {
        }
        frame "CHANNEL_ATTRIBUTE_CO_CTR_TIMEBASE_DIG_FLTR_MIN_PULSE_WIDTH" {
        }
        frame "CHANNEL_ATTRIBUTE_CO_CTR_TIMEBASE_DIG_FLTR_TIMEBASE_RATE" {
        }
        frame "CHANNEL_ATTRIBUTE_AI_VOLTAGE_DB_REF" {
        }
        frame "CHANNEL_ATTRIBUTE_AI_SOUND_PRESSURE_DB_REF" {
        }
        frame "CHANNEL_ATTRIBUTE_AI_ACCEL_DB_REF" {
        }
        frame "CHANNEL_ATTRIBUTE_AO_FUNC_GEN_FREQ" {
        }
        frame "CHANNEL_ATTRIBUTE_AO_FUNC_GEN_AMPLITUDE" {
        }
        frame "CHANNEL_ATTRIBUTE_AO_FUNC_GEN_OFFSET" {
        }
        frame "CHANNEL_ATTRIBUTE_AO_FUNC_GEN_SQUARE_DUTY_CYCLE" {
        }
        frame "CHANNEL_ATTRIBUTE_AO_VOLTAGE_CURRENT_LIMIT" {
        }
        frame "CHANNEL_ATTRIBUTE_AO_FUNC_GEN_FM_DEVIATION" {
        }
        frame "CHANNEL_ATTRIBUTE_DO_OVERCURRENT_LIMIT" {
        }
        frame "CHANNEL_ATTRIBUTE_DO_OVERCURRENT_REENABLE_PERIOD" {
        }
        frame "CHANNEL_ATTRIBUTE_AI_PROBE_ATTEN" {
        }
        frame "CHANNEL_ATTRIBUTE_AI_DC_OFFSET" {
        }
        frame "CHANNEL_ATTRIBUTE_AI_EDDY_CURRENT_PROX_PROBE_SENSITIVITY" {
        }
        frame "CHANNEL_ATTRIBUTE_DI_DIG_FLTR_TIMEBASE_RATE" {
        }
        frame "CHANNEL_ATTRIBUTE_CI_PULSE_FREQ_DIG_FLTR_MIN_PULSE_WIDTH" {
        }
        frame "CHANNEL_ATTRIBUTE_CI_PULSE_FREQ_DIG_FLTR_TIMEBASE_RATE" {
        }
        frame "CHANNEL_ATTRIBUTE_CI_PULSE_TIME_DIG_FLTR_MIN_PULSE_WIDTH" {
        }
        frame "CHANNEL_ATTRIBUTE_CI_PULSE_TIME_DIG_FLTR_TIMEBASE_RATE" {
        }
        frame "CHANNEL_ATTRIBUTE_CI_PULSE_TICKS_DIG_FLTR_MIN_PULSE_WIDTH" {
        }
        frame "CHANNEL_ATTRIBUTE_CI_PULSE_TICKS_DIG_FLTR_TIMEBASE_RATE" {
        }
        frame "CHANNEL_ATTRIBUTE_AI_BRIDGE_SHUNT_CAL_SHUNT_CAL_A_RESISTANCE" {
        }
        frame "CHANNEL_ATTRIBUTE_AI_BRIDGE_SHUNT_CAL_SHUNT_CAL_A_ACTUAL_RESISTANCE" {
        }
        frame "CHANNEL_ATTRIBUTE_AI_BRIDGE_SHUNT_CAL_SHUNT_CAL_B_RESISTANCE" {
        }
        frame "CHANNEL_ATTRIBUTE_AI_BRIDGE_SHUNT_CAL_SHUNT_CAL_B_ACTUAL_RESISTANCE" {
        }
        frame "CHANNEL_ATTRIBUTE_AI_FORCE_IEPE_SENSOR_SENSITIVITY" {
        }
        frame "CHANNEL_ATTRIBUTE_AI_BRIDGE_INITIAL_RATIO" {
        }
        frame "CHANNEL_ATTRIBUTE_AI_BRIDGE_TWO_POINT_LIN_FIRST_ELECTRICAL_VAL" {
        }
        frame "CHANNEL_ATTRIBUTE_AI_BRIDGE_TWO_POINT_LIN_FIRST_PHYSICAL_VAL" {
        }
        frame "CHANNEL_ATTRIBUTE_AI_BRIDGE_TWO_POINT_LIN_SECOND_ELECTRICAL_VAL" {
        }
        frame "CHANNEL_ATTRIBUTE_AI_BRIDGE_TWO_POINT_LIN_SECOND_PHYSICAL_VAL" {
        }
        frame "CHANNEL_ATTRIBUTE_CI_COUNT_EDGES_COUNT_RESET_DIG_FLTR_MIN_PULSE_WIDTH" {
        }
        frame "CHANNEL_ATTRIBUTE_CI_COUNT_EDGES_COUNT_RESET_DIG_FLTR_TIMEBASE_RATE" {
        }
        frame "CHANNEL_ATTRIBUTE_AI_THRMCPL_LEAD_OFFSET_VOLTAGE" {
        }
        frame "CHANNEL_ATTRIBUTE_AI_FILTER_DELAY" {
        }
        frame "CHANNEL_ATTRIBUTE_AI_VELOCITY_IEPE_SENSOR_DB_REF" {
        }
        frame "CHANNEL_ATTRIBUTE_AI_VELOCITY_IEPE_SENSOR_SENSITIVITY" {
        }
        frame "CHANNEL_ATTRIBUTE_AI_ROSETTE_STRAIN_GAGE_ORIENTATION" {
        }
        frame "CHANNEL_ATTRIBUTE_AO_FILTER_DELAY_ADJUSTMENT" {
        }
        frame "CHANNEL_ATTRIBUTE_AI_FILTER_DELAY_ADJUSTMENT" {
        }
        frame "CHANNEL_ATTRIBUTE_AO_FILTER_DELAY" {
        }
        frame "CHANNEL_ATTRIBUTE_CI_DUTY_CYCLE_DIG_FLTR_MIN_PULSE_WIDTH" {
        }
        frame "CHANNEL_ATTRIBUTE_CI_DUTY_CYCLE_DIG_FLTR_TIMEBASE_RATE" {
        }
        frame "CHANNEL_ATTRIBUTE_CI_MAX_MEAS_PERIOD" {
        }
        frame "CHANNEL_ATTRIBUTE_CI_THRESH_VOLTAGE" {
        }
        frame "CHANNEL_ATTRIBUTE_AI_DIG_FLTR_LOWPASS_CUTOFF_FREQ" {
        }
        frame "CHANNEL_ATTRIBUTE_AI_DIG_FLTR_HIGHPASS_CUTOFF_FREQ" {
        }
        frame "CHANNEL_ATTRIBUTE_AI_DIG_FLTR_BANDPASS_CENTER_FREQ" {
        }
        frame "CHANNEL_ATTRIBUTE_AI_DIG_FLTR_BANDPASS_WIDTH" {
        }
        frame "CHANNEL_ATTRIBUTE_AI_DIG_FLTR_NOTCH_CENTER_FREQ" {
        }
        frame "CHANNEL_ATTRIBUTE_AI_DIG_FLTR_NOTCH_WIDTH" {
        }
        frame "CHANNEL_ATTRIBUTE_CI_VELOCITY_LIN_ENCODER_DIST_PER_PULSE" {
        }
        frame "CHANNEL_ATTRIBUTE_CI_VELOCITY_ENCODER_A_INPUT_DIG_FLTR_MIN_PULSE_WIDTH" {
        }
        frame "CHANNEL_ATTRIBUTE_CI_VELOCITY_ENCODER_A_INPUT_DIG_FLTR_TIMEBASE_RATE" {
        }
        frame "CHANNEL_ATTRIBUTE_CI_VELOCITY_ENCODER_B_INPUT_DIG_FLTR_MIN_PULSE_WIDTH" {
        }
        frame "CHANNEL_ATTRIBUTE_CI_VELOCITY_ENCODER_B_INPUT_DIG_FLTR_TIMEBASE_RATE" {
        }
        frame "CHANNEL_ATTRIBUTE_CI_VELOCITY_MEAS_TIME" {
        }
        frame "CHANNEL_ATTRIBUTE_CI_COUNT_EDGES_GATE_DIG_FLTR_MIN_PULSE_WIDTH" {
        }
        frame "CHANNEL_ATTRIBUTE_CI_COUNT_EDGES_GATE_DIG_FLTR_TIMEBASE_RATE" {
        }
        frame "CHANNEL_ATTRIBUTE_AI_ACCEL_CHARGE_SENSITIVITY" {
        }
        frame "CHANNEL_ATTRIBUTE_AI_ACCEL_4_WIRE_DC_VOLTAGE_SENSITIVITY" {
        }
        frame "CHANNEL_ATTRIBUTE_AI_DATA_XFER_MAX_RATE" {
        }
        frame "CHANNEL_ATTRIBUTE_AI_SENSOR_POWER_VOLTAGE" {
        }
        frame "CHANNEL_ATTRIBUTE_AI_FILTER_FREQ" {
        }
        frame "CHANNEL_ATTRIBUTE_AI_INPUT_LIMITS_FAULT_DETECT_UPPER_LIMIT" {
        }
        frame "CHANNEL_ATTRIBUTE_AI_INPUT_LIMITS_FAULT_DETECT_LOWER_LIMIT" {
        }
        frame "CHANNEL_ATTRIBUTE_CI_FREQ_THRESH_VOLTAGE" {
        }
        frame "CHANNEL_ATTRIBUTE_CI_FREQ_HYST" {
        }
        frame "CHANNEL_ATTRIBUTE_CI_PERIOD_THRESH_VOLTAGE" {
        }
        frame "CHANNEL_ATTRIBUTE_CI_PERIOD_HYST" {
        }
        frame "CHANNEL_ATTRIBUTE_CI_COUNT_EDGES_THRESH_VOLTAGE" {
        }
        frame "CHANNEL_ATTRIBUTE_CI_COUNT_EDGES_HYST" {
        }
        frame "CHANNEL_ATTRIBUTE_CI_COUNT_EDGES_COUNT_DIR_THRESH_VOLTAGE" {
        }
        frame "CHANNEL_ATTRIBUTE_CI_COUNT_EDGES_COUNT_DIR_HYST" {
        }
        frame "CHANNEL_ATTRIBUTE_CI_COUNT_EDGES_COUNT_RESET_THRESH_VOLTAGE" {
        }
        frame "CHANNEL_ATTRIBUTE_CI_COUNT_EDGES_COUNT_RESET_HYST" {
        }
        frame "CHANNEL_ATTRIBUTE_CI_COUNT_EDGES_GATE_THRESH_VOLTAGE" {
        }
        frame "CHANNEL_ATTRIBUTE_CI_COUNT_EDGES_GATE_HYST" {
        }
        frame "CHANNEL_ATTRIBUTE_CI_FILTER_FREQ" {
        }
        frame "CHANNEL_ATTRIBUTE_CI_FILTER_DELAY" {
        }
        frame "CHANNEL_ATTRIBUTE_AO_FUNC_GEN_START_PHASE" {
        }
        frame "CHANNEL_ATTRIBUTE_AO_COMMON_MODE_OFFSET" {
        }
        frame "CHANNEL_ATTRIBUTE_PWR_VOLTAGE_SETPOINT" {
        }
        frame "CHANNEL_ATTRIBUTE_PWR_CURRENT_SETPOINT" {
        }
      }
      n9 = Unbundle By Name(w10) -> ("code"=w11:i32)
      n10 = Bundle By Name(cluster=T1 {"status"=0, "value"=0.0} ("Message Data out"), "value"=w8, "status"=w11) -> (w7:T1)
    }
    frame Error {
    }
  }
  "error out" <- w5
  "Task map out" <- w3
  "Message Data out" <- w1
